vi "Timestamp from dat file.vi"(10 "dat file path":path) -> (2 "time stamp":timestamp)   [LabVIEW 2018]
uses:
  <vilib>/Utility/miscctls.llb/LVDateTimeRec.ctl
  <vilib>/regexp/Match Regular Expression.xnode
panel:
  in  "date time rec":T1
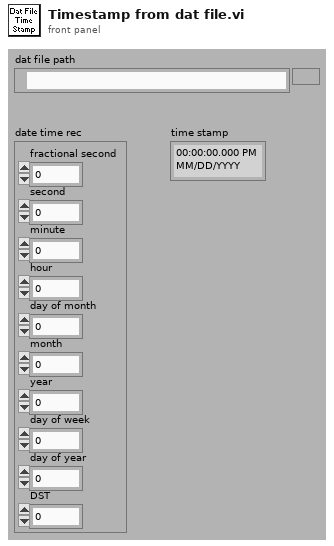
[diagram p1: front panel]
types:
  T1 = typedef "LVDateTimeRec.ctl" = cluster{"fractional second":dbl, "second":i32, "minute":i32, "hour":i32, "day of month":i32, "month":i32, "year":i32, "day of week":i32, "day of year":i32, "DST":i32}
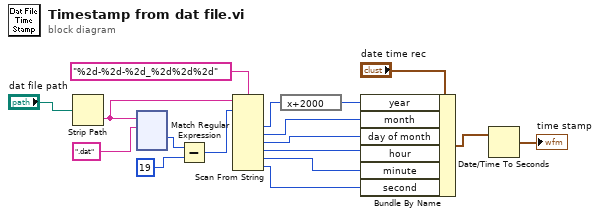
[diagram p0: block diagram]
diagram:
  n1 = Strip Path(path="dat file path") -> (name=w13:string)  [unwired: 1 out]
  n2 = xnode "Match Regular Expression"("input string"=w13, "regular expression"=".dat") -> ("offset past match"=w16:i32)  [unwired: 4 in, 4 out]
  n3 = Subtract(x=w16, y=19) -> (x-y=w14:i32)
  n4 = Scan From String(format string="%2d-%2d-%2d_%2d%2d%2d", input string=w13, initial scan location=w14) -> (output 1=w10:i32, output 2=w8:i32, output 3=w7:i32, output 4=w6:i32, output 5=w5:i32, output 6=w4:i32)  [unwired: 7 in, 3 out]
  n5 = expression code="x+2000"(w10) -> (w9:i32)
  n6 = Bundle By Name(cluster="date time rec", "year"=w9, "month"=w8, "day of month"=w7, "hour"=w6, "minute"=w5, "second"=w4) -> (w3:T1)
  n7 = Date/Time To Seconds(2:w3) -> (0:→"time stamp":timestamp)  [unwired: 1 in]
